vi "Main.vi"() -> ()   [LabVIEW 2014]
uses:
  <vilib>/Utility/miscctls.llb/LVPoint32TypeDef.ctl
  <vilib>/Utility/miscctls.llb/LVRowAndColumnTypeDef.ctl
  <vilib>/Utility/error.llb/DialogType.ctl
  Subs/G-signal.vi
panel:
  in  "合格率:":dbl format="%#_g%%"
  in  "合格数:":dbl
  in  "总测试数:":dbl
  in  "托盘料满？":bool=TRUE
  out "MES字符串":string
  out "2~100":string
  out "错误输出":errorcluster
  in  "错误输入":errorcluster caption="错误输入（无错误）"
  out "状态":string
  out "托盘ID":string
  out "架子ID":string
  out "LOT NO.":string
  out "作业员ID":string
  out "机器名":string
  out "线别":string
  out "坐标":T1
  in  "多列列表框 2":i32[](listbox)
  in  "运行时间":string
  out "PLC":bool
  out "SR700":bool
  out "SR2000-2":bool
  out "SR2000-1":bool
  in  "Auto?":bool
  out "Pass/NG":bool
  in  "MES":bool
  in  "PLC I/O监视":bool
  in  "退出":bool
  in  "配置":bool caption="cog_edit"
  in  "开始":bool
  in  "多列列表框":i32[](listbox)
  in  "Exit":bool
  out "Error Out":errorcluster
  out "Error Report":string
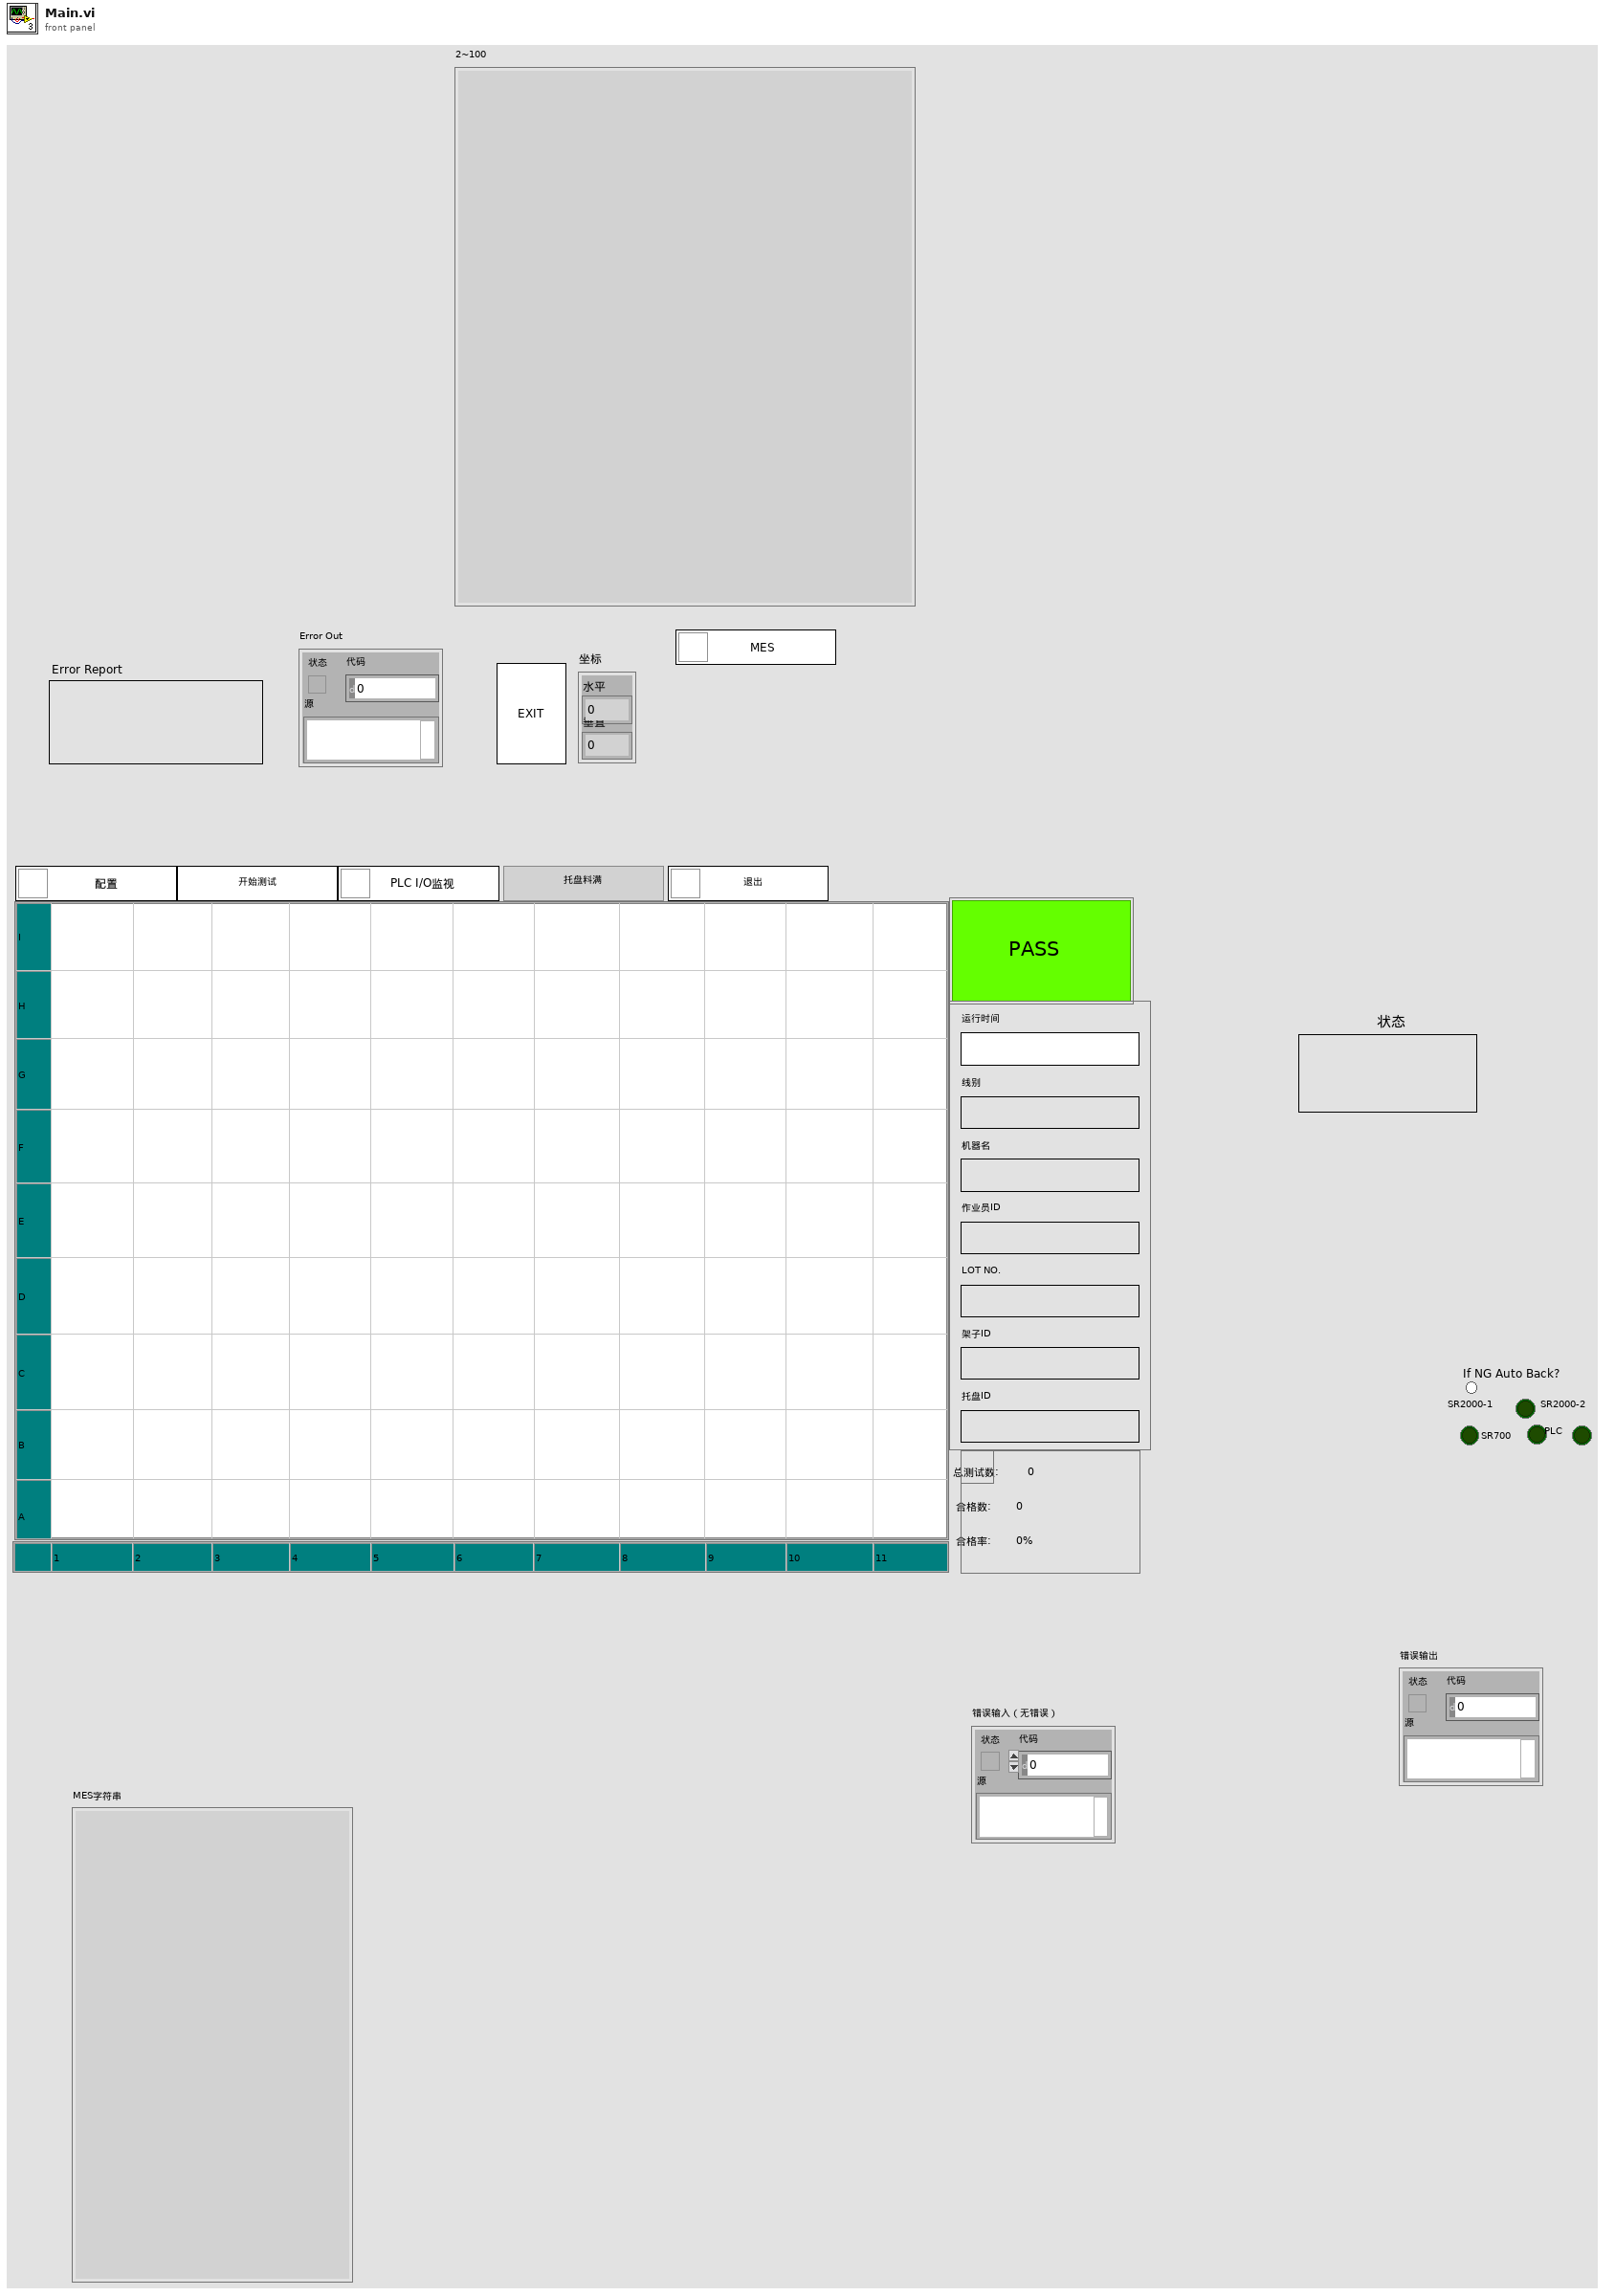
[diagram p1: front panel]
types:
  T1 = typedef "LVPoint32TypeDef.ctl" = cluster{"Horizontal":i32, "Vertical":i32}
  T2 = cluster{"Case Name":string, "Case Data":string}[]
  T3 = typedef "全局参数.ctl" = cluster{"串口设置":cluster{"PLC端口":string, "扫描端口RS2000 ":string, "扫描端口RS700 ":string}, "路径 ":cluster{"条码路径":path, "ME路径":path, "配置文件路径":path, "本VI路径":path}, "NG品":cluster{"位置1NG？":bool, "位置2NG？":bool, "基板箱NG？ ":bool}, "config":cluster{"SR2000-1":refnum<vi>, "SR2000-2":refnum<vi>, "PLC":refnum<vi>, "SR700":refnum<vi>, "Auto?":refnum<vi>, "Pass/NG":refnum<vi>, "开始":refnum<vi>, "Quit":refnum<vi>, "运行时间":refnum<vi>, "多列列表框":refnum<vi>, "基板箱到位？ ":bool, "传感器工位1":bool, "传感器工位2":bool, "基板条码OK？":bool, "工位1条码OK？":bool, "工位2条码OK？":bool, "重新测试":refnum<vi>, "状态":refnum<vi>}, "条码字符串":cluster{"工位1字符串":string, "工位2字符串":string, "基板箱字符串":string}, "MES配置":cluster{"线别":string, "机器名称":string, "作业员ID":string, "LOT NO.":string, "架子ID":string, "托盘ID+1":string, "产品ID+X":string, "基板箱ID+时间日期":string}, "MES[]":cluster{"线别名称":string, "LOT NO":string, "机器名":string}[], "启用MES":bool, "MES字符串":string, "判断托盘料吗？":cluster{"工位1逻辑与":bool, "工位2逻辑与":bool, "托盘料满？":bool}}
  T4 = enum8{"Enabled", "Disabled", "Disabled and Grayed Out"}
  T5 = typedef "amc_Message Queue.ctl" = refnum<queue>
  T6 = typedef "LVRowAndColumnTypeDef.ctl" = cluster{"Row":i32, "Column":i32}
  T7 = cluster{"线别名称":string, "LOT NO":string, "机器名":string}[]
  T8 = enum16{"open", "replace", "create", "open or create", "replace or create", "replace or create with confirmation"}
  T9 = cluster{"X0":bool, "X1":bool, "X2":bool, "X3":bool, "X4":bool, "X5":bool, "X6":bool, "X7":bool, "X10":bool, "X11":bool, "X12 门禁A":bool, "X13":bool, "X14":bool, "X15":bool, "X16":bool, "X17":bool}
  T10 = cluster{"Y0":bool, "Y1":bool, "Y2":bool, "Y3":bool, "Y4":bool, "Y5":bool, "Y6":bool, "Y7":bool, "Y10":bool, "Y11":bool, "Y12":bool, "Y13 蜂鸣器":bool, "Y14 基板箱到位":bool, "Y15 到达扫码1":bool, "Y16 到达扫码2":bool, "Y17":bool}
  T11 = cluster{"X0":bool, "X1":bool, "X2":bool, "X3":bool, "X4":bool, "X5":bool, "X6":bool, "X7":bool, "X10":bool, "X11":bool, "X12":bool, "X13":bool, "X14":bool, "X15":bool, "X16":bool, "X17":bool}
  T12 = cluster{"线别名称":string, "LOT NO":string, "机器名":string, "作业员ID":string}
  T13 = cluster{"工位1字符串":string, "工位2字符串":string, "基板箱字符串":string}
  T14 = cluster{"线别":string, "机器名称":string, "作业员ID":string, "LOT NO.":string, "架子ID":string, "托盘ID+1":string, "产品ID+X":string, "基板箱ID+时间日期":string}
  T15 = typedef "DialogType.ctl" = u16
  T16 = enum32{"invalid app kind", "Development System", "Run Time System", "Student Edition", "Embedded LabVIEW", "Evaluation", "Custom"}
  T17 = cluster{"串口设置":cluster{"PLC端口":string, "扫描端口RS2000 ":string, "扫描端口RS700 ":string}, "路径 ":cluster{"条码路径":path, "ME路径":path, "配置文件路径":path, "本VI路径":path}, "NG品":cluster{"位置1NG？":bool, "位置2NG？":bool, "基板箱NG？ ":bool}, "config":cluster{"SR2000-1":refnum<vi>, "SR2000-2":refnum<vi>, "PLC":refnum<vi>, "SR700":refnum<vi>, "Auto?":refnum<vi>, "Pass/NG":refnum<vi>, "开始":refnum<vi>, "Quit":refnum<vi>, "运行时间":refnum<vi>, "多列列表框":refnum<vi>, "基板箱到位？ ":bool, "传感器工位1":bool, "传感器工位2":bool, "基板条码OK？":bool, "工位1条码OK？":bool, "工位2条码OK？":bool}, "条码字符串":cluster{"工位1字符串":string, "工位2字符串":string, "基板箱字符串":string}}
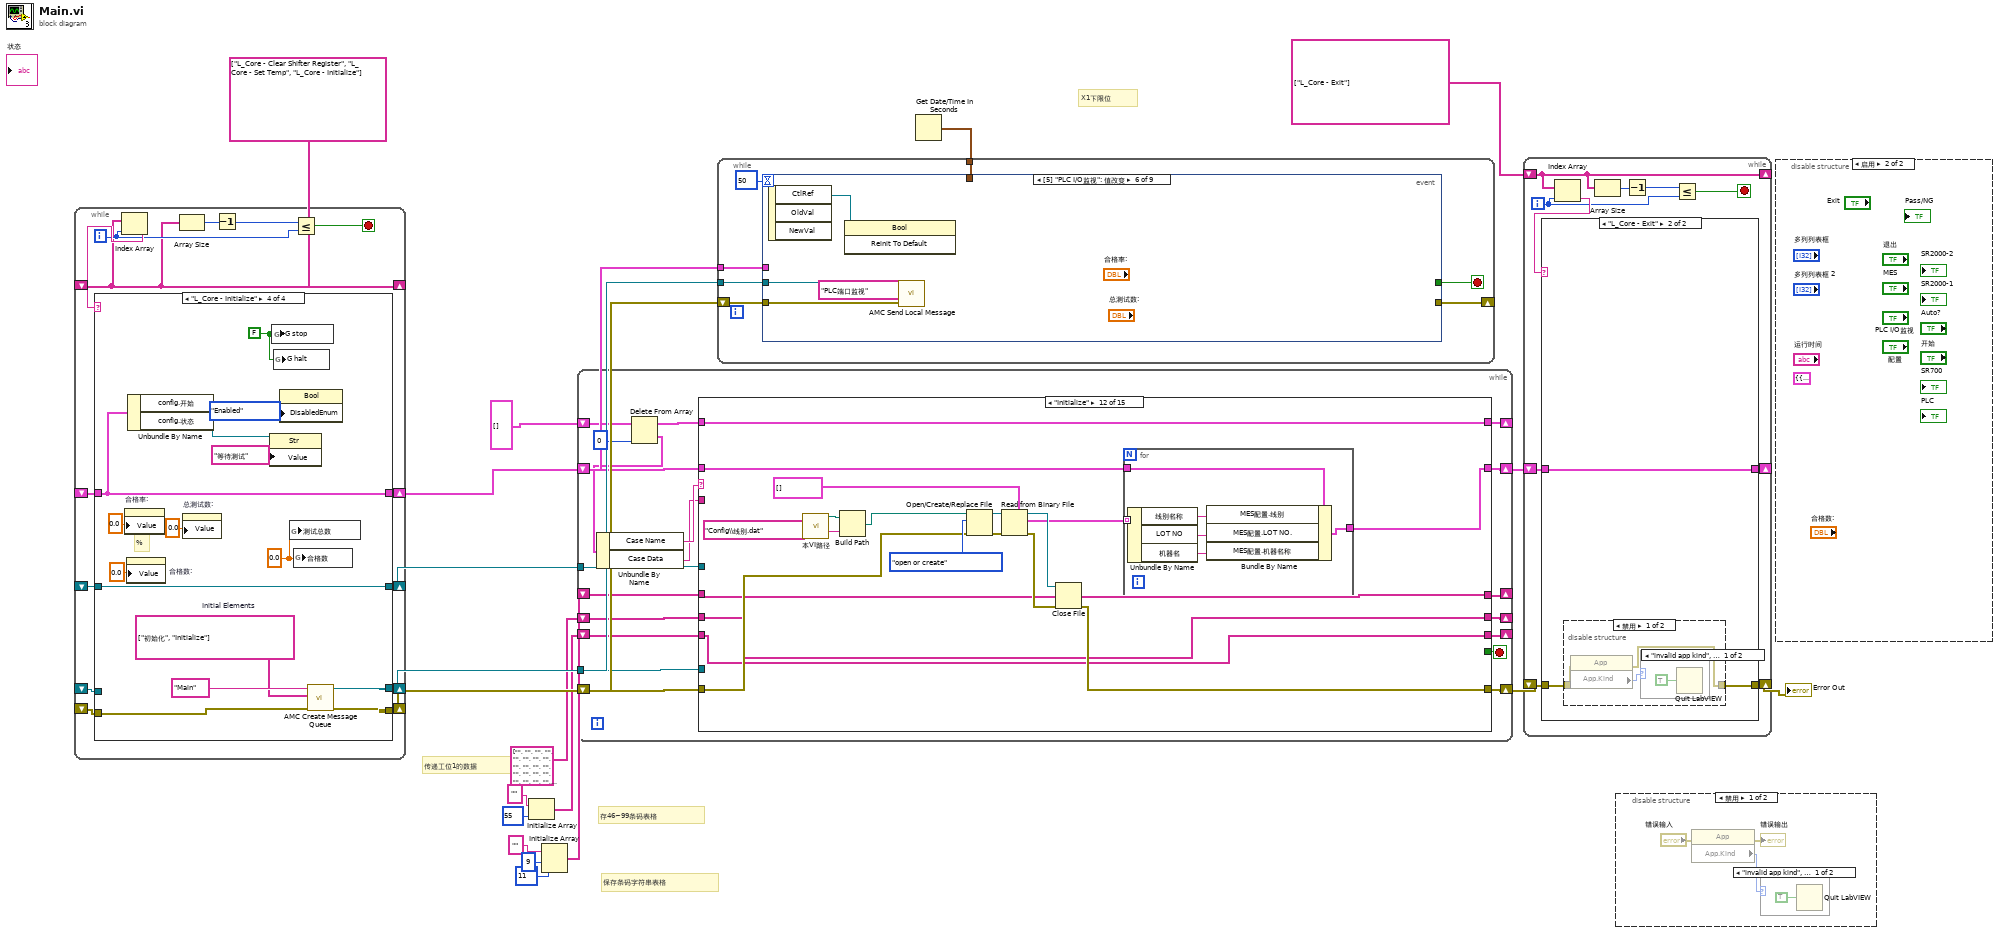
[diagram p0: block diagram]
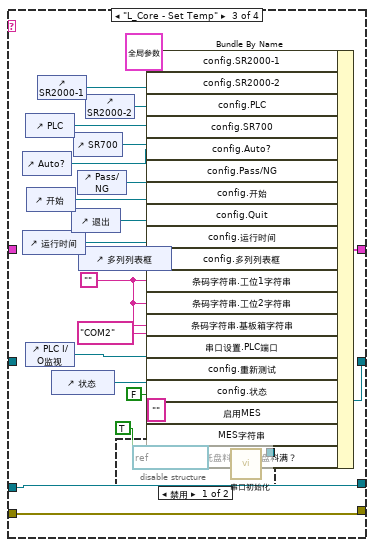
[diagram p10: hidden frame]
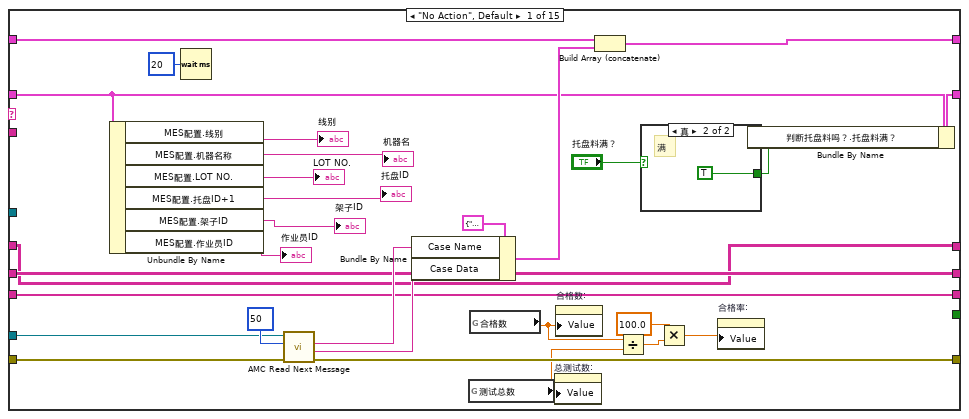
[diagram p12: hidden frame]
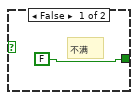
[diagram p13: hidden frame]
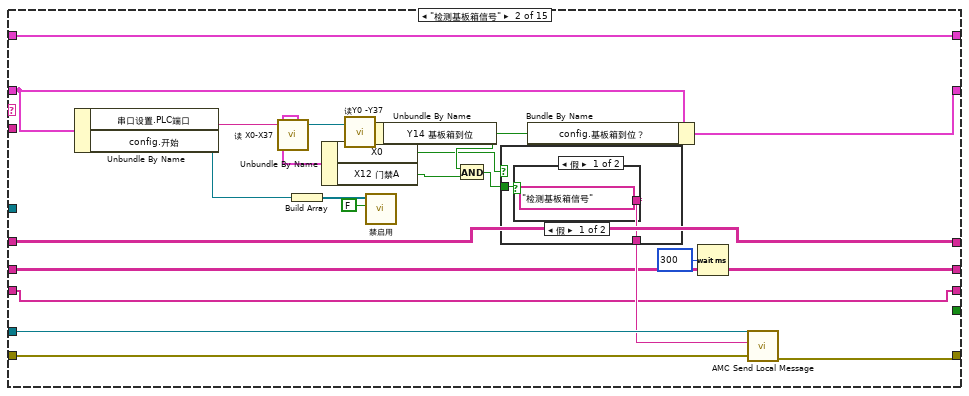
[diagram p14: hidden frame]
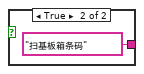
[diagram p15: hidden frame]
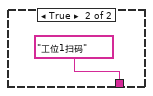
[diagram p16: hidden frame]
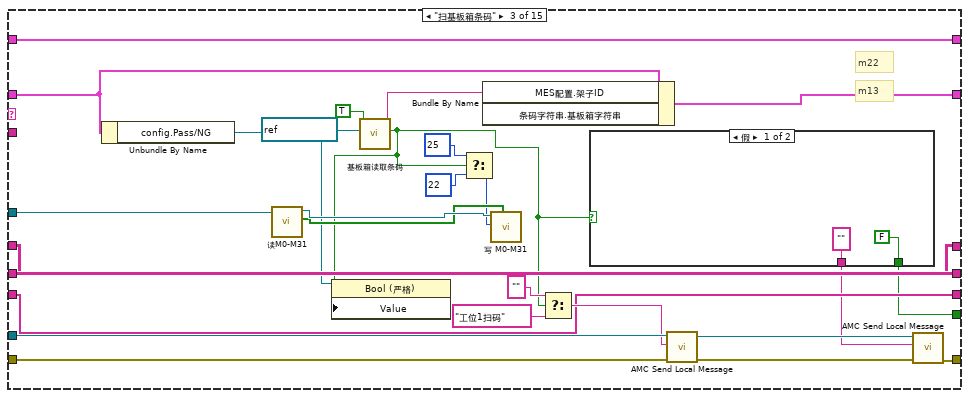
[diagram p17: hidden frame]
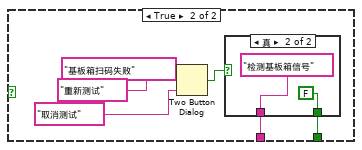
[diagram p18: hidden frame]
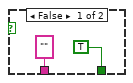
[diagram p19: hidden frame]
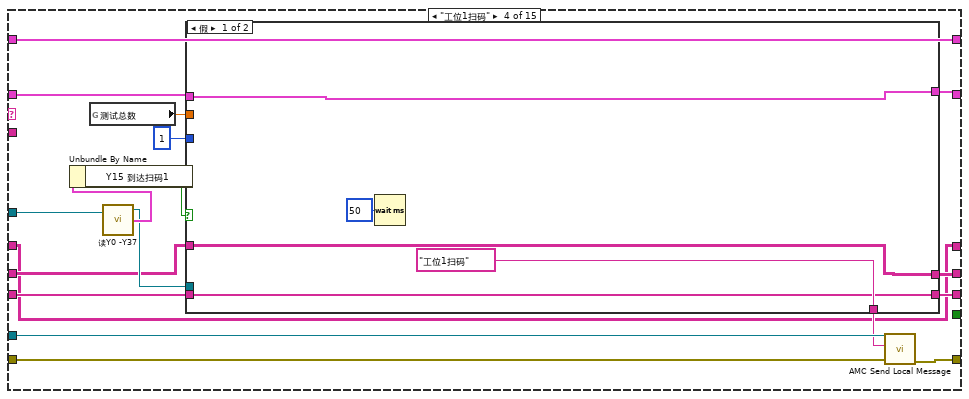
[diagram p20: hidden frame]
diagram:
  # "保存条码字符串表格"
  # "传递工位1的数据"
  # "存46~99条码表格"
  # "X1下限位"
  n1 = while "App INIT" {
    shift-right: [w26] -> _
    shift-left: string[] ["L_Core - Clear Shifter Register", "L_Core - Set Temp", "L_Core - Initialize"] -> [w26]
    shift-right: [w33] -> w18
    shift-left: _ -> [w32]
    shift-right: [w20] -> w11
    shift-left: _ -> [w23]
    shift-right: [w25] -> w12
    shift-left: _ -> [w24]
    shift-right: [w22] -> w9
    shift-left: _ -> [w21]
    i -> [w30]
    stop <- w27 stop-if-true
    n2 = Index Array(array=w26, index=w30) -> (element=w31:string)
    n3 = case shown="\"L_Core - Initialize\"" w31 {
      tunnel: [_ w39 w50 w79] -> w33
      tunnel: w32 -> [_ w39 w50 _]
      tunnel: [w36 w38 w61 w77] -> w25
      tunnel: w24 -> [w36 w38 w61 w76]
      tunnel: w23 -> [w35 w37 _ w68]
      tunnel: [w34 _ w46 w72] -> w22
      tunnel: w21 -> [w34 _ _ w72]
      tunnel: [w35 w37 w60 w68] -> w20
      frame "No Action", Default {
      }
      frame "L_Core - Clear Shifter Register" {
      }
      frame "L_Core - Set Temp" {
        w48 = ""
        n4 = control-ref of="Auto?"() -> (w55:refnum<vi>)
        n5 = control-ref of="运行时间"() -> (w51:refnum<vi>)
        n6 = control-ref of="PLC"() -> (w57:refnum<vi>)
        n7 = control-ref of="PLC I/O监视"() -> (w45:refnum<vi>)
        n8 = control-ref of="开始"() -> (w53:refnum<vi>)
        n9 = control-ref of="SR2000-1"() -> (w59:refnum<vi>)
        n10 = control-ref of="状态"() -> (w44:refnum<vi>)
        n11 = control-ref of="退出"() -> (w52:refnum<vi>)
        n12 = control-ref of="SR700"() -> (w56:refnum<vi>)
        n13 = control-ref of="Pass/NG"() -> (w54:refnum<vi>)
        n14 = control-ref of="多列列表框"() -> (w49:refnum<vi>)
        n15 = control-ref of="SR2000-2"() -> (w58:refnum<vi>)
        n16 = disable-structure shown="禁用" {
          disable-tunnel: [w63 _] -> w46
          frame Disabled {
            n17 = call "串口初始化.vi"("VISA引用句柄输入"=refnum<visa-resource-name> "COM2") -> ("VISA引用句柄输出"=w63:refnum<visa-resource-name>)  [unwired: 9 in, 1 out]
          }
          frame Enabled {
          }
        }
        n18 = Bundle By Name(cluster=T3 {"串口设置"={"PLC端口"="COM1", "扫描端口RS2000 "="", "扫描端口RS700 "=""}, "路径 "={"条码路径"=path "", "ME路径"=path "", "配置文件路径"=path "", "本VI路径"=path ""}, "NG品"={"位置1NG？"=TRUE, "位置2NG？"=TRUE, "基板箱NG？ "=TRUE}, "config"={"SR2000-1"=refnum, "SR2000-2"=refnum, "PLC"=refnum, "SR700"=refnum, "Auto?"=refnum, "Pass/NG"=refnum, "开始"=refnum, "Quit"=refnum, "运行时间"=refnum, "多列列表框"=refnum, "基板箱到位？ "=TRUE, "传感器工位1"=TRUE, "传感器工位2"=TRUE, "基板条码OK？"=FALSE, "工位1条码OK？"=FALSE, "工位2条码OK？"=FALSE, "重新测试"=refnum, "状态"=refnum}, "条码字符串"={"工位1字符串"="", "工位2字符串"="", "基板箱字符串"=""}, "MES配置"={"线别"="", "机器名称"="", "作业员ID"="", "LOT NO."="", "架子ID"="", "托盘ID+1"="", "产品ID+X"="", "基板箱ID+时间日期"=""}, "MES[]"=[], "启用MES"=FALSE, "MES字符串"="", "判断托盘料吗？"={"工位1逻辑与"=TRUE, "工位2逻辑与"=TRUE, "托盘料满？"=TRUE}} ("簇"), "config.SR2000-1"=w59, "config.SR2000-2"=w58, "config.PLC"=w57, "config.SR700"=w56, "config.Auto?"=w55, "config.Pass/NG"=w54, "config.开始"=w53, "config.Quit"=w52, "config.运行时间"=w51, "config.多列列表框"=w49, "条码字符串.工位1字符串"=w48, "条码字符串.工位2字符串"=w48, "条码字符串.基板箱字符串"=w48, "串口设置.PLC端口"="COM2", "config.重新测试"=w45, "config.状态"=w44, "启用MES"=FALSE, "MES字符串"="", "判断托盘料吗？.托盘料满？"=TRUE) -> (w60:T3)
      }
      frame "L_Core - Initialize" {
        w64 = 0.0 ("总测试数")
        w71 = FALSE ("G stop")
        w75 = string[] ["初始化", "Initialize"]  # Initial Elements
        # "%"
        n19 = property on="合格率:" class="DigNum (严格)"("Value"=0.0 ("合格率:")) -> ()  [unwired: 2 in, 2 out]
        n20 = property on="合格数:" class="DigNum (严格)"("Value"=0.0 ("合格数:")) -> ()  [unwired: 2 in, 2 out]
        n21 = Unbundle By Name(w68) -> ("config.开始"=w74:refnum<vi>, "config.状态"=w70:refnum<vi>)
        n22 = property on="总测试数:" class="DigNum (严格)"("Value"=0.0 ("总测试数:")) -> ()  [unwired: 2 in, 2 out]
        n23 = property class="Str"(reference=w70, "Value"="等待测试" ("值")) -> ()  [unwired: 1 in, 2 out]
        n24 = global write "G-signal.vi" "G stop"(w71) -> ()
        n25 = global write "G-signal.vi" "G halt"(w71) -> ()
        n26 = property class="Bool"(reference=w74, "DisabledEnum"=T4."Enabled" ("禁用")) -> ()  [unwired: 1 in, 2 out]
        n27 = global write "G-signal.vi" "测试总数"(w64) -> ()
        n28 = global write "G-signal.vi" "合格数"(w64) -> ()
        n29 = call <userlib>:"AMC Create Message Queue.vi"("error in (no error)"=w76, "Initial Message Names"=w75, "Message Queue Name"="Main") -> ("error out"=w77:errorcluster, "Message Queue out"=w79:T5)  [unwired: 7 in]
      }
    }
    n30 = Array Size(array=w26) -> (size(s)=w29:i32)
    n31 = Decrement(x=w29) -> (x-1=w28:i32)
    n32 = Less Or Equal?(x=w28, y=w30) -> (x <= y?=w27:bool)
  }
  n33 = Initialize Array("", 55 ("维数大小")) -> (w1:string[])
  n34 = Initialize Array("", 9 ("维数大小"), 11 ("维数大小")) -> (w4:string[][])
  n35 = while "Primary Execution Loop" {
    shift-right: [w98] -> w19
    shift-left: w11 -> [w99]
    tunnel: w18 -> [w97]
    shift-right: [w88] -> w15
    shift-left: w12 -> [w96]
    shift-right: [w84] -> _
    shift-left: T2 [] ("Case") -> [w93]
    shift-right: [w87] -> _
    shift-left: string[][] [["", "", "", "", "", "", "", "", "", "", ""], ["", "", "", "", "", "", "", "", "", "", ""], ["", "", "", "", "", "", "", "", "", "", ""], ["", "", "", "", "", "", "", "", "", "", ""], ["", "", "", "", "", "", "", "", "", "", ""], ["", "", "", "", "", "", "", "", "", "", ""], ["", "", "", "", "", "", "", "", "", "", ""], ["", "", "", "", "", "", "", "", "", "", ""], ["", "", "", "", "", "", "", "", "", "", ""]] ("项名") -> [w86]
    tunnel: w9 -> [w85]
    shift-right: [w83] -> _
    shift-left: w1 -> [w82]
    shift-right: [w81] -> _
    shift-left: w4 -> [w80]
    stop <- w95 stop-if-true
    n36 = Delete From Array(array=w93, index=0 ("索引")) -> (deleted portion=w91:cluster{"Case Name":string, "Case Data":string}, array with subset deleted=w92:T2)  [unwired: 1 in]
    n37 = Unbundle By Name(w91) -> ("Case Name"=w90:string, "Case Data"=w89:string)
    n38 = case shown="\"Initialize\"" w90 {
      tunnel: w96 -> [w126 w146 w182 w208 w249 w323 w337 _ w373 w383 w402 w430 w456 w472 w491]
      tunnel: w97 -> [w127 w147 w183 w209 w250 _ w338 _ _ w384 _ _ _ _ w490]
      tunnel: w99 -> [w107 w144 w171 w212 w269 w331 w345 w360 w364 w387 w411 w435 w458 w467 w485]
      tunnel: [w106 w143 w172 w213 w270 w331 w345 w360 w371 w386 w411 w434 w458 w467 w485] -> w98
      tunnel: w92 -> [w123 w152 w163 w214 w271 w328 w347 w359 w374 w390 w403 w432 w455 w469 w488]
      tunnel: [_ _ w158 _ _ _ _ _ _ _ _ _ _ _ TRUE ("NewVal")] -> w95
      tunnel: w89 -> [_ _ _ _ _ _ _ _ _ _ _ _ _ _ _]
      tunnel: [w119 w142 w160 w207 w256 w323 w334 w356 w373 w382 w402 w431 w456 w468 w487] -> w88
      tunnel: [w118 w133 w180 w211 w268 w330 w348 w358 w372 w385 w392 w429 w457 w466 w486] -> w87
      tunnel: w86 -> [w118 w133 w180 w204 w264 w330 w348 w358 w372 w385 w392 w429 w457 w466 w486]
      tunnel: w85 -> [_ _ w184 w202 w266 _ w346 w357 _ _ _ _ _ _ w481]
      tunnel: [w122 w152 w163 w214 w271 w328 w347 w359 w374 w390 w403 w432 w455 w469 w488] -> w84
      tunnel: [w111 w134 w165 w201 w259 w329 w344 w355 w366 w379 w393 w428 w452 w465 w479] -> w83
      tunnel: w82 -> [w111 w134 w165 w200 w262 w329 w344 w355 w366 w379 w393 w428 w452 w465 w479]
      tunnel: [w109 w132 w164 w199 w261 _ w339 w354 w362 w378 w391 w427 w450 w464 w478] -> w81
      tunnel: w80 -> [w109 w132 w164 w199 w260 w327 w339 w354 w362 w378 w391 w427 w451 w464 w478]
      frame "No Action", Default {
        n39 = Unbundle By Name(w107) -> ("MES配置.线别"=→"线别":string, "MES配置.机器名称"=→"机器名":string, "MES配置.LOT NO."=→"LOT NO.":string, "MES配置.托盘ID+1"=→"托盘ID":string, "MES配置.架子ID"=→"架子ID":string, "MES配置.作业员ID"=→"作业员ID":string)
        n40 = Wait (ms)(milliseconds to wait=u32 20 ("等待时间（毫秒）")) -> ()  [unwired: 1 out]
        n41 = call <userlib>:"AMC Read Next Message.vi"("error in (no error)"=w126, "timeout (1ms)"=50, "Message Queue in"=w127) -> ("error out"=w119:errorcluster, "Message Value"=w120:string, "Message Name"=w121:string)  [unwired: 2 in, 4 out]
        n42 = Bundle By Name(cluster=cluster{"Case Name":string, "Case Data":string} {"Case Name"="", "Case Data"=""} ("Case"), "Case Name"=w121, "Case Data"=w120) -> (w124:cluster{"Case Name":string, "Case Data":string})
        n43 = global read "G-signal.vi" "测试总数"() -> (w103:dbl)
        n44 = global read "G-signal.vi" "合格数"() -> (w104:dbl)
        n45 = property on="总测试数:" class="DigNum (严格)"("Value"=w103) -> ()  [unwired: 2 in, 2 out]
        n46 = property on="合格数:" class="DigNum (严格)"("Value"=w104) -> ()  [unwired: 2 in, 2 out]
        n47 = Build Array (concatenate)(w123, w124) -> (w122:T2)
        n48 = Divide(x=w104, y=w103) -> (x/y=w102:dbl)
        n49 = case shown="真" "托盘料满？" {
          tunnel: [FALSE TRUE] -> w105
          frame False {
            # "不满"
          }
          frame True {
            # "满"
          }
        }
        n50 = Multiply(x=100.0, y=w102) -> (x*y=w100:dbl)
        n51 = property on="合格率:" class="DigNum (严格)"("Value"=w100) -> ()  [unwired: 2 in, 2 out]
        n52 = Bundle By Name(cluster=w107, "判断托盘料吗？.托盘料满？"=w105) -> (w106:T3)
      }
      frame "检测基板箱信号" {
        n53 = Unbundle By Name(w144) -> ("串口设置.PLC端口"=w151:string, "config.开始"=w135:refnum<vi>)
        n54 = call "读 X0-X37.vi"("VISA资源名称"=w151) -> ("X0-X17"=w149:T9, "VISA资源名称输出"=w141:refnum<visa-resource-name>)  [unwired: 5 in, 2 out]
        n55 = Build Array(w135) -> (w136:refnum<vi>[])
        n56 = Unbundle By Name(w149) -> ("X0"=w131:bool, "X12 门禁A"=w148:bool)
        n57 = call "读Y0 -Y37.vi"("VISA资源名称"=w141) -> ("Y0-Y17"=w150:T10)  [unwired: 6 in, 2 out]
        n58 = call "禁启用.vi"("Enabled？"=FALSE, "数组"=w136) -> ()  [unwired: 10 in]
        n59 = Unbundle By Name ("基板箱到位")(w150) -> ("Y14 基板箱到位"=w140:bool)
        n60 = And(x=w140, y=w148) -> (x .and. y?=w138:bool)
        n61 = case shown="假" w131 {
          tunnel: [w153 "工位1扫码" ("Message Name")] -> w145
          tunnel: w138 -> [w154 _]
          frame False {
            n62 = case shown="假" w154 {
              tunnel: ["检测基板箱信号" "扫基板箱条码" ("Message Name")] -> w153
              frame False {
              }
              frame True {
              }
            }
          }
          frame True {
          }
        }
        n63 = Bundle By Name(cluster=w144, "config.基板箱到位？"=w140) -> (w143:T3)
        n64 = Wait (ms)(milliseconds to wait=u32 300 ("等待时间（毫秒）")) -> ()  [unwired: 1 out]
        n65 = call <userlib>:"AMC Send Local Message.vi"("error in (no error)"=w146, "Message Name"=w145, "Message Queue in"=w147) -> ("error out"=w142:errorcluster)  [unwired: 7 in, 1 out]
      }
      frame "扫基板箱条码" {
        # "m13"
        # "m22"
        n66 = Unbundle By Name(w171) -> ("config.Pass/NG"=w170:refnum<vi>)
        n67 = call "读M0-M31.vi"("VISA资源名称"=w184) -> ("M"=w178:bool[], "VISA资源名称输出"=w179:refnum<visa-resource-name>)  [unwired: 8 in, 1 out]
        n68 = call "基板箱读取条码.vi"("开启条码?"=TRUE, "VISA resource name"=refnum<visa-resource-name> "COM1") -> ("基板箱条码"=w166:string, "基板箱NG？"=w167:bool)  [unwired: 7 in]
        n69 = property class="Bool (严格)"(reference=w170, "Value"=w167) -> ()  [unwired: 1 in, 2 out]
        n70 = Select(t=25 ("索引"), s=w167, f=22 ("索引")) -> (s? t:f=w175:i32)
        n71 = Bundle By Name(cluster=w171, "MES配置.架子ID"=w166, "条码字符串.基板箱字符串"=w166) -> (w172:T3)
        n72 = call "写 M0-M31.vi"("Old VAL"=w178, "索引"=w175, "VISA资源名称"=w179) -> ()  [unwired: 8 in, 1 out]
        n73 = Select(t="" ("地址"), s=w167, f="工位1扫码" ("地址")) -> (s? t:f=w181:string)
        n74 = case shown="假" w167 {
          tunnel: ["" w188] -> w159
          tunnel: [FALSE w187] -> w158
          frame False {
          }
          frame True {
            n75 = Two Button Dialog(message="基板箱扫码失败" ("消息"), 1:"取消测试" ("F按钮名称（“取消”）"), 2:"重新测试" ("T按钮名称（“确定”）")) -> (T button?=w189:bool)
            n76 = case shown="真" w189 {
              tunnel: ["" "检测基板箱信号"] -> w188
              tunnel: [TRUE FALSE] -> w187
              frame False {
              }
              frame True {
              }
            }
          }
        }
        n77 = call <userlib>:"AMC Send Local Message.vi"("error in (no error)"=w182, "Message Name"=w181, "Message Queue in"=w183) -> ("error out"=w161:errorcluster, "Message Queue out"=w162:T5)  [unwired: 7 in]
        n78 = call <userlib>:"AMC Send Local Message.vi"("error in (no error)"=w161, "Message Name"=w159, "Message Queue in"=w162) -> ("error out"=w160:errorcluster)  [unwired: 7 in, 1 out]
      }
      frame "工位1扫码" {
        n79 = global read "G-signal.vi" "测试总数"() -> (w198:dbl)
        n80 = call "读Y0 -Y37.vi"("VISA资源名称"=w202) -> ("VISA资源名称输出"=w205:refnum<visa-resource-name>, "Y0-Y17"=w210:T10)  [unwired: 6 in, 1 out]
        n81 = Unbundle By Name(w210) -> ("Y15 到达扫码1"=w203:bool)
        n82 = case shown="假" w203 {
          tunnel: [w216 w244] -> w213
          tunnel: w212 -> [w216 w243]
          tunnel: [w218 w232] -> w211
          tunnel: ["工位1扫码" w228] -> w206
          tunnel: w205 -> [_ w238]
          tunnel: w204 -> [w218 _]
          tunnel: [w215 w229] -> w201
          tunnel: w200 -> [w215 _]
          tunnel: w198 -> [_ w221]
          tunnel: 1 -> [_ w220]
          frame False {
            n83 = Wait (ms)(milliseconds to wait=u32 50 ("等待时间（毫秒）")) -> ()  [unwired: 1 out]
          }
          frame True {
            # "布尔为真代表有NG"
            n84 = Add(x=w221, y=w220) -> (x+y=w222:dbl)
            n85 = Unbundle By Name(w243) -> ("config.多列列表框"=w236:refnum<vi>, "config.Pass/NG"=w237:refnum<vi>)
            n86 = global write "G-signal.vi" "测试总数"(w222) -> ()
            n87 = call "test.vi"("COLUMN"=9, "ROW"=6, "引用"=w236) -> ("料盘ID NG？"=w225:bool, "条码1"=w232:string[][], "条码字符串"=w231:string, "托盘ID"=w233:string, "工位一NG?"=w230:bool, "46~99条码数组"=w229:string[], "工位1逻辑与"=w226:bool)  [unwired: 1 in]
            n88 = case shown="真" w225 {
              tunnel: [0 _] -> w224
              frame False {
              }
              frame True {
                n89 = One Button Dialog(message="托盘ID扫码错误" ("消息"), button name ("OK")="确定" ("按钮名称（“确定”）")) -> ()  [unwired: 1 out]
              }
            }
            n90 = property class="Bool (严格)"(reference=w237, "Value"=w230) -> ()  [unwired: 1 in, 2 out]
            n91 = Bundle By Name(cluster=w243, "条码字符串.工位1字符串"=w231, "NG品.位置1NG？"=w230, "MES配置.托盘ID+1"=w233, "判断托盘料吗？.工位1逻辑与"=w226) -> (w244:T3)
            n92 = call "读M0-M31.vi"("VISA资源名称"=w238) -> ("M"=w241:bool[], "VISA资源名称输出"=w242:refnum<visa-resource-name>)  [unwired: 8 in, 1 out]
            n93 = Select(t=23 ("索引"), s=FALSE, f=20 ("索引")) -> (s? t:f=w227:i32)
            n94 = call "写 M0-M31.vi"("Old VAL"=w241, "索引"=w227, "VISA资源名称"=w242) -> ()  [unwired: 8 in, 1 out]
            n95 = flat-sequence {
              tunnel: ["工位2扫码" ("f")] -> w228
              tunnel: w224 -> [_]
              frame #0 {
              }
            }
          }
        }
        n96 = call <userlib>:"AMC Send Local Message.vi"("error in (no error)"=w208, "Message Name"=w206, "Message Queue in"=w209) -> ("error out"=w207:errorcluster)  [unwired: 7 in, 1 out]
      }
      frame "工位2扫码" {
        # "Y6为假时代表料盘扫码OK"
        n97 = call "读Y0 -Y37.vi"("VISA资源名称"=w266) -> ("VISA资源名称输出"=w265:refnum<visa-resource-name>, "Y0-Y17"=w267:T10)  [unwired: 6 in, 1 out]
        n98 = Unbundle By Name(w267) -> ("Y16 到达扫码2"=w263:bool)
        n99 = case shown="真" w263 {
          tunnel: [w278 w313] -> w270
          tunnel: w269 -> [w278 w297]
          tunnel: [w279 _] -> w268
          tunnel: ["工位2扫码" w312] -> w254
          tunnel: w265 -> [_ w303]
          tunnel: w264 -> [w279 w307]
          tunnel: w262 -> [w276 w300]
          tunnel: [w277 w299] -> w261
          tunnel: w260 -> [w277 _]
          tunnel: [w276 _] -> w259
          tunnel: ["" "保存报表"] -> w255
          tunnel: ["" w285] -> w251
          frame False {
            n100 = Wait (ms)(milliseconds to wait=u32 50 ("等待时间（毫秒）")) -> ()  [unwired: 1 out]
          }
          frame True {
            # "21为前进"
            # "下限位"
            n101 = Unbundle By Name(w297) -> ("判断托盘料吗？.托盘料满？"=w289:bool, "NG品.位置1NG？"=w292:bool, "config.多列列表框"=w308:refnum<vi>, "config.Pass/NG"=w305:refnum<vi>, "判断托盘料吗？.工位1逻辑与"=w284:bool)
            n102 = call "读X0-X37.vi"("VISA资源名称"=w303) -> ("X0-X17"=w302:T11, "VISA资源名称输出"=w295:refnum<visa-resource-name>, "错误输出"=w298:errorcluster)  [unwired: 5 in, 1 out]
            n103 = flat-sequence {
              tunnel: w298 -> [w320]
              tunnel: [w320] -> _
              frame #0 {
                n104 = Wait (ms)(milliseconds to wait=u32 100 ("等待时间（毫秒）")) -> ()  [unwired: 1 out]
              }
            }
            n105 = Unbundle By Name(w302) -> ("X1"=w301:bool)
            n106 = case shown="假" w301 {
              tunnel: ["工位1扫码" ("f") "检测基板箱信号" ("f")] -> w290
              frame False {
              }
              frame True {
              }
            }
            n107 = call "工位2扫码.vi"("工位1逻辑与"=w284, "工位1表格"=w307, "46~99编号数组"=w300, "MulticolumnListbox输入"=w308) -> ("有空料？"=w287:bool, "条码字符串"=w306:string, "工位2NG?"=w291:bool, "1~99保存报表"=w299:string[][])  [unwired: 4 in]
            n108 = Not(x=w291) -> (.not. x?=w293:bool)
            n109 = Not(x=w292) -> (.not. x?=w294:bool)
            n110 = And(x=w294, y=w293) -> (x .and. y?=w288:bool)
            n111 = property class="Bool (严格)"(reference=w305, "Value"=w291) -> ()  [unwired: 1 in, 2 out]
            n112 = global read "G-signal.vi" "合格数"() -> (w280:dbl)
            n113 = call "托盘料满状态判断.vi"("有空料？"=w287, "全盘料满？"=w288, "托盘料满？"=w289) -> ("OK？"=w283:bool, "数值"=w286:i32)  [unwired: 7 in]
            n114 = case shown="真" w283 {
              tunnel: ["" "生成MES条码"] -> w285
              tunnel: 1 -> [_ w317]
              tunnel: w280 -> [_ w315]
              frame False {
              }
              frame True {
                n115 = Add(x=w317, y=w315) -> (x+y=w316:dbl)
                n116 = global write "G-signal.vi" "合格数"(w316) -> ()
              }
            }
            n117 = Not(x=w283) -> (.not. x?=w282:bool)
            n118 = Not(x=w291) -> (.not. x?=w304:bool)
            n119 = Select(t="Halt", s=w282, f=w290) -> (s? t:f=w312:string)
            n120 = Bundle By Name(cluster=w297, "条码字符串.工位2字符串"=w306, "NG品.位置2NG？"=w291, "config.工位2条码OK？"=w304) -> (w313:T3)
            n121 = call "读M0-M31.vi"("VISA资源名称"=w295) -> ("M"=w309:bool[], "VISA资源名称输出"=w310:refnum<visa-resource-name>)  [unwired: 8 in, 1 out]
            n122 = call "写 M0-M31.vi"("Old VAL"=w309, "索引"=w286, "VISA资源名称"=w310) -> ()  [unwired: 8 in, 1 out]
          }
        }
        n123 = call <userlib>:"AMC Send Local Message.vi"("error in (no error)"=w249, "Message Name"=w251, "Message Queue in"=w250) -> ("error out"=w252:errorcluster, "Message Queue out"=w253:T5)  [unwired: 7 in]
        n124 = call <userlib>:"AMC Send Local Message.vi"("error in (no error)"=w252, "Message Name"=w254, "Message Queue in"=w253) -> ("error out"=w257:errorcluster, "Message Queue out"=w258:T5)  [unwired: 7 in]
        n125 = call <userlib>:"AMC Send Local Message.vi"("error in (no error)"=w257, "Message Name"=w255, "Message Queue in"=w258) -> ("error out"=w256:errorcluster)  [unwired: 7 in, 1 out]
      }
      frame "保存报表" {
        n126 = call "Path 2.vi"() -> ("appended path"=w325:path)  [unwired: 11 in]
        n127 = call "保存报表.vi"("数组"=w327, "条码"="99条码保存", "当前VI路径"=w325) -> ()  [unwired: 9 in]
        n128 = Wait (ms)(milliseconds to wait=u32 100 ("等待时间（毫秒）")) -> ()  [unwired: 1 out]
      }
      frame "Halt" {
        # "进板感应"
        n129 = disable-structure shown="启用" {
          disable-tunnel: w346 -> [w351 _]
          frame Disabled {
            n130 = call "读X0-X37.vi"("VISA资源名称"=w351) -> ("X0-X17"=w350:T11)  [unwired: 5 in, 3 out]
            n131 = Unbundle By Name(w350) -> ()  [unwired: 1 out]
          }
          frame Enabled {
          }
        }
        n132 = Two Button Dialog(message="工位2测试失败上传MES？" ("消息"), 1:"不上传" ("F按钮名称（“取消”）"), 2:"上传" ("T按钮名称（“确定”）")) -> (T button?=w340:bool)
        n133 = case shown="真" w340 {
          tunnel: ["" "生成MES条码"] -> w332
          frame False {
          }
          frame True {
          }
        }
        n134 = call <userlib>:"AMC Send Local Message.vi"("error in (no error)"=w337, "Message Name"=w332, "Message Queue in"=w338) -> ("error out"=w335:errorcluster, "Message Queue out"=w336:T5)  [unwired: 7 in]
        n135 = flat-sequence {
          tunnel: ["工位1扫码"] -> w333
          tunnel: w332 -> [_]
          frame #0 {
          }
        }
        n136 = call <userlib>:"AMC Send Local Message.vi"("error in (no error)"=w335, "Message Name"=w333, "Message Queue in"=w336) -> ("error out"=w334:errorcluster)  [unwired: 7 in, 1 out]
      }
      frame "PLC端口监视" {
        n137 = call "编程口协议.vi"("串口号"=w357) -> ("错误输出"=w356:errorcluster)  [unwired: 9 in, 1 out]
      }
      frame "MES配置" {
        n138 = Unbundle By Name(w364) -> ("启用MES"=w365:bool)
        n139 = call "系统配置.vi"() -> ("线别配置 2"=w370:T12)  [unwired: 11 in]
        n140 = Unbundle By Name(w370) -> ("线别名称"=w369:string, "LOT NO"=w368:string, "机器名"=w367:string, "作业员ID"=w363:string)
        n141 = Bundle By Name(cluster=w364, "MES配置.线别"=w369, "MES配置.LOT NO."=w368, "MES配置.机器名称"=w367, "启用MES"=w365, "MES配置.作业员ID"=w363) -> (w371:T3)
        n142 = Wait (ms)(milliseconds to wait=u32 500 ("等待时间（毫秒）")) -> ()  [unwired: 1 out]
      }
      frame "生成MES条码" {
        n143 = call <userlib>:"AMC Send Local Message.vi"("error in (no error)"=w383, "Message Name"="END", "Message Queue in"=w384) -> ("error out"=w382:errorcluster)  [unwired: 7 in, 1 out]
        n144 = Unbundle By Name(w387) -> ("条码字符串"=w389:T13, "MES配置"=w388:T14)
        n145 = Wait (ms)(milliseconds to wait=u32 500 ("等待时间（毫秒）")) -> ()  [unwired: 1 out]
        n146 = call "2~100条码ID.vi"("MES配置输入"=w388, "条码字符串输入"=w389) -> ("时间"=w376:string, "MES字符串"=w375:string, "1-99"=w377:string)  [unwired: 7 in]
        "2~100" <- w377
        "MES字符串" <- w375
        n147 = Bundle By Name(cluster=w387, "MES字符串"=w375, "MES配置.产品ID+X"=w377, "MES配置.基板箱ID+时间日期"=w376) -> (w386:T3)
      }
      frame "初始化" {
        n148 = Unbundle By Name(w411) -> ("config.多列列表框"=w410:refnum<vi>, "config.Pass/NG"=w401:refnum<vi>, "config.开始"=w397:refnum<vi>, "config.重新测试"=w394:refnum<vi>)  [unwired: 1 out]
        n149 = property class="MCListbox (严格)"(reference=w410, "SelMode"=0 ("选择模式")) -> (reference out=w407:refnum<vi>)  [unwired: 1 in, 1 out]
        n150 = property class="Bool (严格)"(reference=w401, "Value"=FALSE) -> ()  [unwired: 1 in, 2 out]
        n151 = Build Array(w397) -> (w399:refnum<vi>[])
        n152 = Build Array(w394) -> (w395:refnum<vi>[])
        n153 = call "禁启用.vi"("Enabled？"=TRUE, "数组"=w399) -> ()  [unwired: 10 in]
        n154 = call "禁启用.vi"("Enabled？"=TRUE, "数组"=w395) -> ()  [unwired: 10 in]
        n155 = for {
          N: 9 -> [_]
          tunnel: w407 -> [w415]
          tunnel: T6 {"Row"=0, "Column"=0} ("活动单元格:活动单元格") -> [w414]
          tunnel: [w412] -> w405
          i -> [w413]
          n156 = for {
            N: 12 -> [_]
            tunnel: w415 -> [w423]
            tunnel: w414 -> [w422]
            tunnel: w413 -> [w420]
            tunnel: [w418] -> w412
            i -> [w419]
            n157 = Bundle By Name(cluster=w422, "Row"=w420, "Column"=w419) -> (w421:T6)
            n158 = property class="MCListbox (严格)"(reference=w423, "ActiveCell"=w421, "CellBG"=u32 13816530) -> (reference out=w418:refnum<vi>)  [unwired: 1 in, 1 out]
          }
        }
        n159 = property class="MCListbox (严格)"(reference=w405, "ItemNames"=string[][] [] ("项名")) -> ()  [unwired: 1 in, 2 out]
      }
      frame "Initialize" {
        n160 = call "本VI路径.vi"() -> ("stripped path"=w426:path)  [unwired: 11 in]
        n161 = Build Path(base path=w426, name or relative path="Config\\线别.dat" ("名称或相对路径")) -> (appended path=w424:path)
        n162 = Open/Create/Replace File(file path (use dialog)=w424, error in=w430, operation (0:open)=T8."open or create" ("操作(0:open)")) -> (refnum out=w441:refnum<file>, error out=w439:errorcluster)  [unwired: 3 in, 1 out]
        n163 = Read from Binary File(5:T7 [], 8:w439, 11:w441) -> (0:w436:errorcluster, 2:w433:T7, 3:w437:refnum<file>)  [unwired: 3 in, 1 out]
        n164 = Close File(refnum=w437, error in=w436) -> (error out=w431:errorcluster)  [unwired: 1 out]
        n165 = for {
          tunnel: w435 -> [w447]
          tunnel: [w446] -> w434
          tunnel: w433 -> [w445] mode=indexing
          n166 = Unbundle By Name(w445) -> ("线别名称"=w444:string, "LOT NO"=w443:string, "机器名"=w442:string)
          n167 = Bundle By Name(cluster=w447, "MES配置.线别"=w444, "MES配置.LOT NO."=w443, "MES配置.机器名称"=w442) -> (w446:T3)
        }
      }
      frame "END" {
        n168 = Unbundle By Name(w458) -> ("MES字符串"=w453:string, "MES配置"=w448:T14)
        n169 = case shown="真" TRUE {
          tunnel: TRUE -> [_ w463]
          tunnel: w453 -> [_ w462]
          tunnel: w451 -> [w459 w460]
          tunnel: w448 -> [_ w461]
          tunnel: [w459 w460] -> w450
          frame False {
          }
          frame True {
            # "上传MES"
            n170 = call "MES操作函数H.vi"("MES字符串"=w462, "总结果（测试）"=w463, "MES配置"=w461) -> ()  [unwired: 8 in, 1 out]
          }
        }
      }
      frame "Error" {
        w474 = T15 0 items=["no dialog", "OK message", "continue or stop message", "OK message + warnings", "continue/stop + warnings"] ("type of dialog (OK msg:1)")
        w475 = T15 2 items=["no dialog", "OK message", "continue or stop message", "OK message + warnings", "continue/stop + warnings"] ("type of dialog (OK msg:1)")
        n171 = Unbundle By Name(w472) -> ("source"=w477:string)
        n172 = call <vilib>:"Simple Error Handler.vi"("type of dialog (OK msg:1)"=w474, "error in (no error)"=w472) -> ("error out"=w473:errorcluster, "message"=w471:string)  [unwired: 3 in, 3 out]
        n173 = Concatenate Strings(w477, w471) -> (→"Error Report":string)
        n174 = call <vilib>:"Simple Error Handler.vi"("type of dialog (OK msg:1)"=w475, "error in (no error)"=w473) -> ("error out"=w476:errorcluster)  [unwired: 3 in, 4 out]
        n175 = call <vilib>:"Clear Errors.vi"("error in (no error)"=w476) -> ("error out"=w468:errorcluster)  [unwired: 5 in, 1 out]
      }
      frame "Exit", "退出" {
        n176 = call <userlib>:"AMC Destroy Message Queue.vi"("error in (no error)"=w491, "Message Queue in"=w490) -> ("error out"=w487:errorcluster)  [unwired: 8 in, 1 out]
        n177 = VISA Close(VISA resource name=w481) -> (error out=w480:errorcluster)  [unwired: 1 in]
        n178 = call <vilib>:"Clear Errors.vi"("error in (no error)"=w480) -> ()  [unwired: 5 in, 2 out]
        n179 = Unbundle By Name(w485) -> ("config.开始"=w482:refnum<vi>)
        n180 = Build Array(w482) -> (w483:refnum<vi>[])
        n181 = call "禁启用.vi"("Enabled？"=TRUE, "数组"=w483) -> ()  [unwired: 10 in]
      }
    }
  }
  n182 = Get Date/Time In Seconds() -> (seconds since 1Jan1904=w13:timestamp)
  n183 = while "Event Handler Loop" {
    tunnel: w18 -> [w497]
    shift-right: [w494] -> _
    shift-left: w12 -> [w495]
    tunnel: w13 -> [w493]
    tunnel: w11 -> [w492]
    stop <- w498 stop-if-true
    n184 = event shown="[5] \"PLC I/O监视\": 值改变" {
      selector: _ -> [_ _ _ _ _ _ _ _ _]
      dyn-events: _ -> [_ _ _ _ _ _ _ _ _]
      timeout: 50 -> [_ _ _ _ _ _ _ _ _]
      tunnel: [w508 _ TRUE ("NewVal") FALSE ("NewVal") _ _ TRUE w542 w552] -> w498
      tunnel: w497 -> [w502 _ w524 w529 w531 w535 w541 w547 w550]
      tunnel: w495 -> [w501 w519 w521 w526 w532 w534 w540 w546 w549]
      tunnel: [w501 w519 w520 w525 _ _ w539 w545 w548] -> w494
      tunnel: w493 -> [w506 _ _ _ _ _ _ _ _]
      tunnel: w492 -> [w504 w513 _ _ _ _ _ _ _]
      event Timeout {
        n185 = event-data() -> ()  [unwired: 2 out]
        n186 = Unbundle By Name(w504) -> ("config.运行时间"=w503:refnum<vi>, "config.状态"=w499:refnum<vi>)
        n187 = Get Date/Time In Seconds() -> (seconds since 1Jan1904=w507:timestamp)
        n188 = Subtract(x=w507, y=w506) -> (x-y=w505:dbl)
        n189 = call "数值值时间字符串.vi"("数值"=w505, "String输入"=w503) -> ()  [unwired: 10 in]
        n190 = property class="Str"(reference=w499, "Value"="等待扫码" ("值")) -> ()  [unwired: 1 in, 2 out]
        n191 = Not A Number/Path/Refnum?(number/path/refnum=w502) -> (NaN/Path/Refnum?=w508:bool)
      }
      event Mouse Move {
        n192 = event-data() -> ("Coords"=w516:T1)  [unwired: 5 out]
        "坐标" <- w516
        n193 = Unbundle By Name(w516) -> ("Horizontal"=w510:i32, "Vertical"=w518:i32)
        n194 = Greater?(x=w510, y=620 ("x")) -> (0:w515:bool)
        n195 = Less?(x=w518, y=35) -> (x < y?=w514:bool)
        n196 = Unbundle By Name(w513) -> ("config.Quit"=w512:refnum<vi>)
        n197 = And(x=w515, y=w514) -> (x .and. y?=w511:bool)
        n198 = property class="Bool"(reference=w512, "Visible"=w511) -> ()  [unwired: 1 in, 2 out]
      }
      event "Exit": Value Change {
        n199 = event-data() -> ()  [unwired: 2 out]
        n200 = call <userlib>:"AMC Send Local Message.vi"("error in (no error)"=w521, "Message Name"="Exit", "Message Queue in"=w524) -> ("error out"=w520:errorcluster)  [unwired: 7 in, 1 out]
      }
      event "开始": Value Change {
        n201 = event-data() -> ()  [unwired: 4 out]
        n202 = call <userlib>:"AMC Send Local Message.vi"("error in (no error)"=w526, "Message Name"="检测基板箱信号", "Message Queue in"=w529) -> ("error out"=w525:errorcluster)  [unwired: 7 in, 1 out]
      }
      event "配置": Value Change {
        n203 = event-data() -> ()  [unwired: 4 out]
        n204 = call <userlib>:"AMC Send Local Message.vi"("error in (no error)"=w532, "Message Name"="MES配置", "Message Queue in"=w531) -> ()  [unwired: 7 in, 2 out]
      }
      event "PLC I/O监视": Value Change {
        n205 = event-data() -> ("CtlRef"=w536:refnum<vi>)  [unwired: 3 out]
        n206 = invoke class="Bool" method="Reinit To Default"(reference=w536) -> ()  [unwired: 2 in, 3 out]
        n207 = call <userlib>:"AMC Send Local Message.vi"("error in (no error)"=w534, "Message Name"="PLC端口监视", "Message Queue in"=w535) -> ()  [unwired: 7 in, 2 out]
      }
      event "退出": Value Change {
        n208 = event-data() -> ()  [unwired: 4 out]
        n209 = call <userlib>:"AMC Send Local Message.vi"("error in (no error)"=w540, "Message Name"="Exit", "Message Queue in"=w541) -> ("error out"=w539:errorcluster)  [unwired: 7 in, 1 out]
      }
      event Menu Selection (User) {
        n210 = event-data() -> ("ItemTag"=w544:string)  [unwired: 1 out]
        n211 = call <userlib>:"AMC Send Local Message.vi"("error in (no error)"=w546, "Message Name"=w544, "Message Queue in"=w547) -> ("error out"=w545:errorcluster)  [unwired: 7 in, 1 out]
        n212 = Equal?(x=w544, y="退出") -> (x = y?=w542:bool)
      }
      event Panel Close? {
        w552 = TRUE  # Discard?
        n213 = event-data() -> ()  [unwired: 5 out]
        n214 = call <userlib>:"AMC Send Local Message.vi"("error in (no error)"=w549, "Message Name"="Exit", "Message Queue in"=w550) -> ("error out"=w548:errorcluster)  [unwired: 7 in, 1 out]
        n215 = event-data("Discard?"=w552) -> ()  [unwired: 1 in, 1 out]
      }
    }
  }
  n216 = while "App Close" {
    shift-right: [w555] -> _
    shift-left: string[] ["L_Core - Exit"] -> [w555]
    shift-right: [w561] -> _
    shift-left: w19 -> [w562]
    shift-right: [w553] -> w8
    shift-left: w15 -> [w554]
    i -> [w557]
    stop <- w556 stop-if-true
    n217 = Index Array(array=w555, index=w557) -> (element=w558:string)
    n218 = case shown="\"L_Core - Exit\"" w558 {
      tunnel: [w564 w567] -> w561
      tunnel: w562 -> [w564 w567]
      tunnel: w554 -> [w563 w566]
      tunnel: [w563 w565] -> w553
      frame "No Action", Default {
      }
      frame "L_Core - Exit" {
        n219 = disable-structure shown="禁用" {
          disable-tunnel: w566 -> [w569 _]
          disable-tunnel: [w568 _] -> w565
          frame Disabled {
            n220 = property class="App"(error in=w569) -> (error out=w568:errorcluster, "App.Kind"=w570:T16)  [unwired: 1 in, 1 out]
            n221 = case shown="\"invalid app kind\", 默认" w570 {
              frame "invalid app kind", Default {
                n222 = Quit LabVIEW(quit? (T)=TRUE ("退出？(T)")) -> ()
              }
              frame "Development System" {
              }
            }
          }
          frame Enabled {
          }
        }
      }
    }
    n223 = Array Size(array=w555) -> (size(s)=w560:i32)
    n224 = Decrement(x=w560) -> (x-1=w559:i32)
    n225 = Less Or Equal?(x=w559, y=w557) -> (x <= y?=w556:bool)
  }
  "Error Out" <- w8
  n226 = disable-structure shown="禁用" {
    frame Disabled {
      n227 = property class="App"(error in="错误输入") -> (error out=→"错误输出":errorcluster, "App.Kind"=w574:T16)  [unwired: 1 in, 1 out]
      n228 = case shown="\"invalid app kind\", 默认" w574 {
        frame "invalid app kind", Default {
          n229 = Quit LabVIEW(quit? (T)=TRUE ("退出？(T)")) -> ()
        }
        frame "Development System" {
        }
      }
    }
    frame Enabled {
    }
  }
  n230 = disable-structure shown="启用" {
    frame Disabled {
    }
    frame Enabled {
      (unwired) T17 {"串口设置"={"PLC端口"="", "扫描端口RS2000 "="", "扫描端口RS700 "=""}, "路径 "={"条码路径"=path "", "ME路径"=path "", "配置文件路径"=path "", "本VI路径"=path ""}, "NG品"={"位置1NG？"=FALSE, "位置2NG？"=FALSE, "基板箱NG？ "=FALSE}, "config"={"SR2000-1"=refnum, "SR2000-2"=refnum, "PLC"=refnum, "SR700"=refnum, "Auto?"=refnum, "Pass/NG"=refnum, "开始"=refnum, "Quit"=refnum, "运行时间"=refnum, "多列列表框"=refnum, "基板箱到位？ "=FALSE, "传感器工位1"=FALSE, "传感器工位2"=FALSE, "基板条码OK？"=FALSE, "工位1条码OK？"=FALSE, "工位2条码OK？"=FALSE}, "条码字符串"={"工位1字符串"="", "工位2字符串"="", "基板箱字符串"=""}}
    }
  }
